vi "MonitoreoSerialDeFlujo.vi"() -> ()   [LabVIEW 2015]
doc: "This VI will continuously monitor the serial port and extract the temperature reading from the received string. This is stored in an array and displayed on the Graph. Press STOP to close the serial port and end the program.\n\nThis program is designed to work with the May 2009 version of the Arduino Temperature program which sends a header, the raw A/D value and the temperature as a float text value.\n\nSelect the appropriate COM port before running this VI. Leave the other serial port settings at their default values (9600, 8, none, 1.0, none)."
uses:
  <vilib>/Instr/_visa.llb/VISA Configure Serial Port (Instr).vi
  <vilib>/MakerHub/LINX/LMH-LINX.lvlib
panel:
  in  "Tiempo de Muestreo":string(combo)
  in  "BaudRate":i32(ring)=10 items=["9600"=9600, "19200"=19200, "38400"=38400, "57600"=57600, "74880"=74880, "115200"=115200]
  in  "Jump Button 4":bool
  in  "Guardar datos a excel":bool
  in  "Rango de grafica":i16(knob) scale=0.0..100.0
  out "FLUJO DE ENTRADA":i32 caption="L/min."
  out "Flujo de entrada y salida":cluster{dbl[], dbl[]}[](graph)
  out "TIEMPO DE MUESTREO":dbl caption="s"
  in  "Jump Button 3":bool
  out "VOLUMEN 1 (L)":i32 caption="L"
  in  "Puerto":refnum<visa-resource-name>="COM3"
  in  "stop":bool
  # "MONITOREO DE SENSORES DE FLUJO YF-S201"
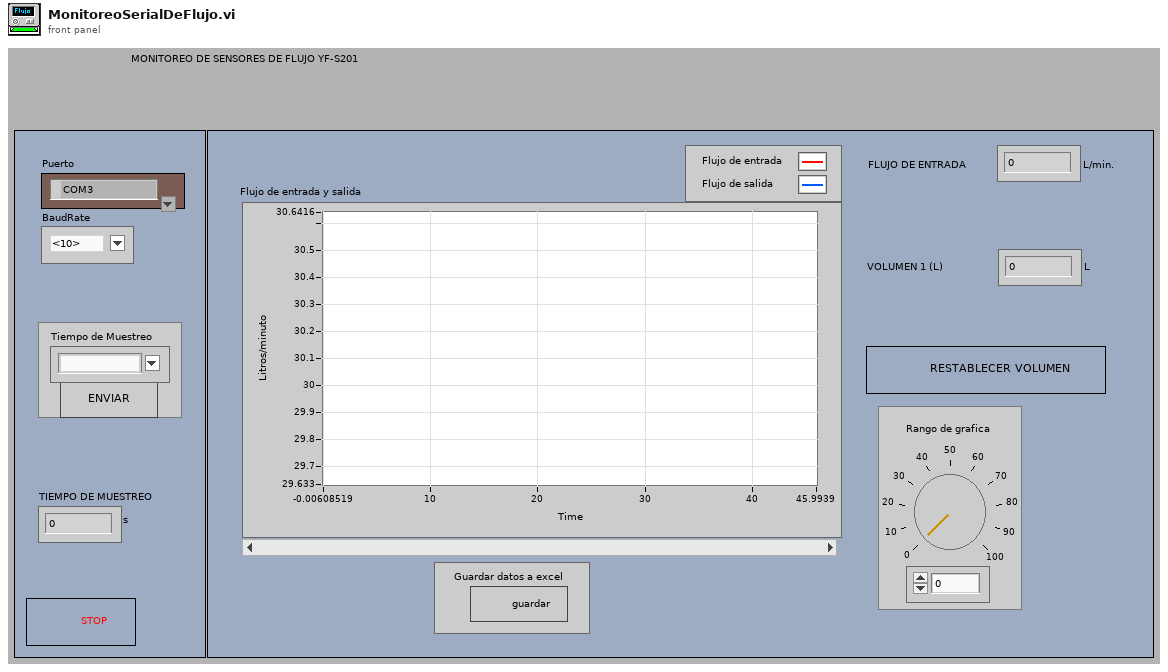
[diagram p1: front panel]
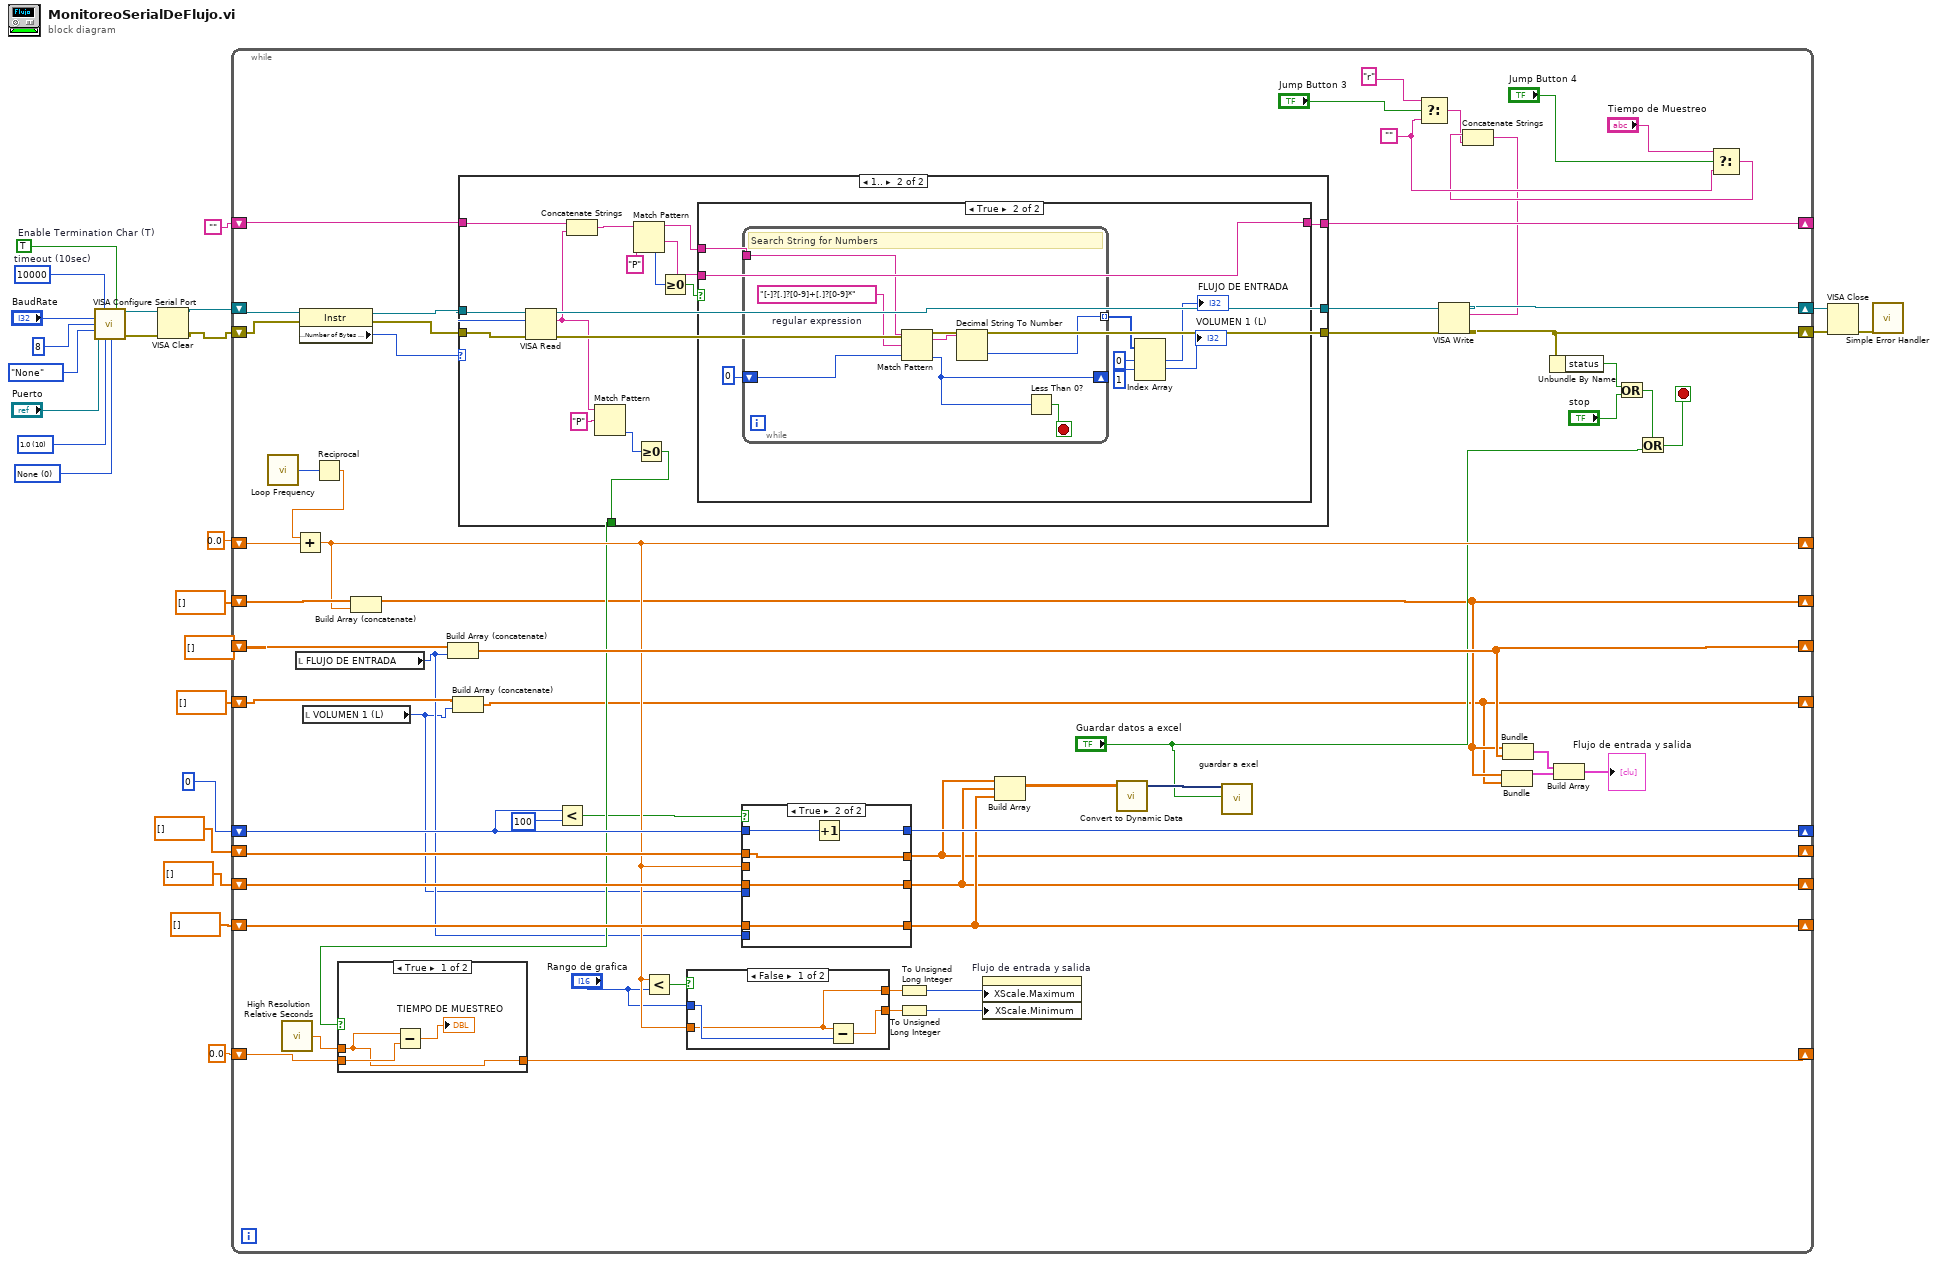
[diagram p0: block diagram]
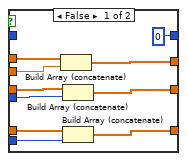
[diagram p2: hidden frame]
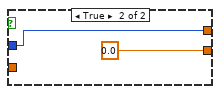
[diagram p3: hidden frame]
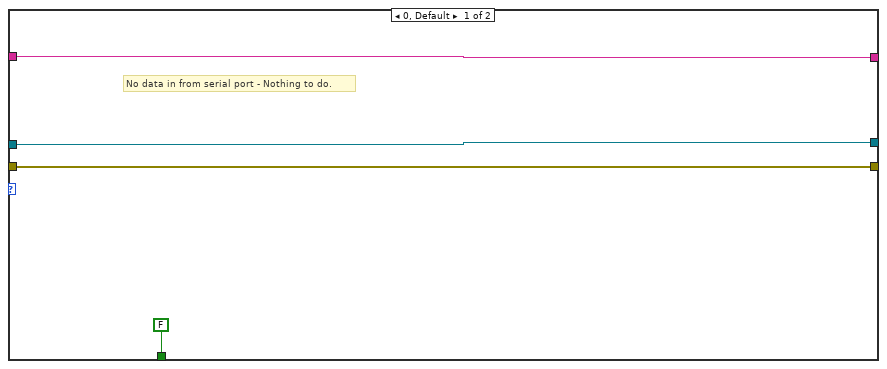
[diagram p5: hidden frame]
diagram:
  w16 = u16 10 items=["1.0"=10, "1.5"=15, "2.0"=20] ("stop bits (10: 1 bit)")
  w17 = u16 0 items=["None", "XON/XOFF", "RTS/CTS", "XON/XOFF & RTS/CTS", "DTR/DSR", "XON/XOFF & DTR/DSR"] ("flow control (0:none)")
  w22 = TRUE  # Enable Termination Char (T)
  w23 = u32 10000  # timeout (10sec)
  n1 = call-poly "VISA Configure Serial Port"("VISA resource name"="Puerto", "timeout (10sec)"=w23, "Enable Termination\nChar (T)"=w22, "baud rate (9600)"="BaudRate", "data bits (8)"=u16 8 ("Data bits (8)"), "parity (0:none)"=enum16{"None", "Odd", "Even", "Mark", "Space"}."None" ("Parity (0:none)"), "stop bits (10: 1 bit)"=w16, "flow control (0:none)"=w17) -> ("VISA resource name out"=w20:refnum<visa-resource-name>, "error out"=w21:errorcluster)  [unwired: 6 in]
  n2 = VISA Clear(VISA resource name=w20, error in (no error)=w21) -> (VISA resource name out=w19:refnum<visa-resource-name>, error out=w3:errorcluster)
  n3 = while {
    shift-right: [w79] -> _
    shift-left: "" -> [w82]
    shift-right: [w27] -> _
    shift-left: dbl[] [] -> [w73]
    shift-right: [w50] -> _
    shift-left: 0.0 -> [w74]
    shift-right: [w61] -> _
    shift-left: dbl[] [] -> [w71]
    shift-right: [w26] -> _
    shift-left: dbl[] [] -> [w72]
    shift-right: [w69] -> _
    shift-left: 0.0 ("relative seconds") -> [w70]
    shift-right: [w56] -> _
    shift-left: 0 -> [w57]
    shift-right: [w51] -> _
    shift-left: dbl[] [] -> [w54]
    shift-right: [w52] -> _
    shift-left: dbl[] [] -> [w53]
    shift-right: [w49] -> _
    shift-left: dbl[] [] -> [w55]
    shift-right: [w76] -> w25
    shift-left: w3 -> [w44]
    shift-right: [w43] -> w2
    shift-left: w19 -> [w84]
    stop <- w60 stop-if-true
    w41 = ""
    n4 = call <vilib>:"Loop Frequency.vi"() -> ("Loop Rate (Hz)"=w64:u32)
    n5 = call <vilib>:"High Resolution Relative Seconds.vi"() -> ("relative seconds"=w65:dbl)
    n6 = local read "FLUJO DE ENTRADA"() -> (w42:i32)
    n7 = property class="Instr"(reference=w84, error in=w44) -> (reference out=w86:refnum<visa-resource-name>, error out=w85:errorcluster, "Serial Settings:Number of Bytes at Serial Port"=w83:u32)
    n8 = local read "VOLUMEN 1 (L)"() -> (w28:i32)
    n9 = Reciprocal(x=w64) -> (1/x=w68:dbl)
    n10 = Add(x=w68, y=w74) -> (x+y=w50:dbl)
    n11 = Build Array (concatenate)(w73, w50) -> (w27:dbl[])
    n12 = Build Array (concatenate)(w71, w42) -> (w61:dbl[])
    n13 = Build Array (concatenate)(w72, w28) -> (w26:dbl[])
    n14 = case shown="1.." w83 {
      selector: w83 -> [_ w126]
      tunnel: [w113 w131] -> w77
      tunnel: [w114 w130] -> w78
      tunnel: w86 -> [w114 w129]
      tunnel: w85 -> [w113 w128]
      tunnel: w82 -> [w112 w127]
      tunnel: [w112 w121] -> w79
      tunnel: [FALSE w115] -> w45
      frame 0, Default {
        # "No data in from serial port - Nothing to do."
      }
      frame 1.. {
        n15 = VISA Read(VISA resource name=w129, byte count=w126, error in (no error)=w128) -> (VISA resource name out=w130:refnum<visa-resource-name>, read buffer=w117:string, error out=w131:errorcluster)  [unwired: 1 out]
        n16 = Concatenate Strings(w127, w117) -> (w120:string)
        n17 = Match Pattern(string=w117, regular expression="P") -> (offset past match=w116:i32)  [unwired: 1 in, 3 out]
        n18 = Match Pattern(string=w120, regular expression="P") -> (before substring=w119:string, after substring=w122:string, offset past match=w124:i32)  [unwired: 1 in, 1 out]
        n19 = Greater Or Equal To 0?(x=w116) -> (x >= 0?=w115:bool)
        n20 = Greater Or Equal To 0?(x=w124) -> (x >= 0?=w123:bool)
        n21 = case shown="True" w123 {
          tunnel: w122 -> [_ w140]
          tunnel: [w132 w140] -> w121
          tunnel: w119 -> [w132 w138]
          frame False {
          }
          frame True {
            n22 = while {
              shift-left: 0 -> [w145]
              shift-right: [w143] -> _
              tunnel: [w147] -> w135 mode=indexing
              tunnel: w138 -> [w141]
              stop <- w146 stop-if-true
              w142 = "[-]?[.]?[0-9]+[.]?[0-9]*"  # regular expression
              # "Search String for Numbers"
              n23 = Match Pattern(string=w141, regular expression=w142, offset (0)=w145) -> (match substring=w144:string, offset past match=w143:i32)  [unwired: 2 out]
              n24 = Decimal String To Number(string=w144) -> (number=w147:i32)  [unwired: 2 in, 1 out]
              n25 = Less Than 0?(x=w143) -> (x < 0?=w146:bool)
            }
            n26 = Index Array(array=w135, index #1=0 ("index"), index #2=1 ("index")) -> (element #1=→"FLUJO DE ENTRADA":i32, element #2=→"VOLUMEN 1 (L)":i32)  [unwired: 1 in, 1 out]
          }
        }
      }
    }
    n27 = case shown="True" w45 {
      tunnel: w70 -> [w109 w110]
      tunnel: w65 -> [w107 _]
      tunnel: [w107 w110] -> w69
      frame True {
        n28 = Subtract(x=w107, y=w109) -> (x-y=→"TIEMPO DE MUESTREO":dbl)
      }
      frame False {
      }
    }
    n29 = Less?(x=w57, y=u32 100) -> (x < y?=w29:bool)
    n30 = Less?(x=w50, y="Rango de grafica") -> (x < y?=w63:bool)
    n31 = case shown="False" w63 {
      tunnel: "Rango de grafica" -> [w103 w105]
      tunnel: [w102 w105] -> w34
      tunnel: [w104 0.0] -> w32
      tunnel: w50 -> [w102 _]
      frame False {
        n32 = Subtract(x=w102, y=w103) -> (x-y=w104:dbl)
      }
      frame True {
      }
    }
    n33 = case shown="True" w29 {
      tunnel: w57 -> [_ w101]
      tunnel: [u32 0 w100] -> w56
      tunnel: w55 -> [w95 w97]
      tunnel: w28 -> [w93 _]
      tunnel: [w96 w99] -> w51
      tunnel: w54 -> [w94 w99]
      tunnel: w42 -> [w91 _]
      tunnel: w53 -> [w92 w98]
      tunnel: [w90 w98] -> w52
      tunnel: [w89 w97] -> w49
      tunnel: w50 -> [w88 _]
      frame False {
        n34 = Build Array (concatenate)(w95, w88) -> (w89:dbl[])
        n35 = Build Array (concatenate)(w94, w93) -> (w96:dbl[])
        n36 = Build Array (concatenate)(w92, w91) -> (w90:dbl[])
      }
      frame True {
        n37 = Increment(x=w101) -> (x+1=w100:u32)
      }
    }
    n38 = To Unsigned Long Integer(number=w34) -> (unsigned 32bit integer=w33:u32)
    n39 = To Unsigned Long Integer(number=w32) -> (unsigned 32bit integer=w31:u32)
    n40 = property on="Flujo de entrada y salida" class="XYGraph (strict)"("XScale.Maximum"=w33, "XScale.Minimum"=w31) -> ()  [unwired: 2 in, 2 out]
    n41 = Build Array(w49, w51, w52) -> (w47:dbl[][])
    n42 = call "Convert to Dynamic Data"("2D Array"=w47) -> ("Dynamic Data Type"=w48:dynamicdata)  [unwired: 3 in]
    n43 = call "guardar a exel"("Signals"=w48, "Enable"="Guardar datos a excel") -> ()  [unwired: 15 in, 3 out]
    n44 = Select(t="r", s="Jump Button 3", f=w41) -> (s? t:f=w38:string)
    n45 = Bundle(w27, w26) -> (w66:cluster{dbl[], dbl[]})  [unwired: 1 in]
    n46 = Bundle(w27, w61) -> (w67:cluster{dbl[], dbl[]})  [unwired: 1 in]
    n47 = Build Array(w67, w66) -> (→"Flujo de entrada y salida":cluster{dbl[], dbl[]}[])
    n48 = Select(t="Tiempo de Muestreo", s="Jump Button 4", f=w41) -> (s? t:f=w39:string)
    n49 = Concatenate Strings(w39, w38) -> (w36:string)
    n50 = VISA Write(VISA resource name=w78, write buffer=w36, error in (no error)=w77) -> (VISA resource name out=w43:refnum<visa-resource-name>, error out=w76:errorcluster)  [unwired: 1 out]
    n51 = Unbundle By Name(w76) -> ("status"=w81:bool)
    n52 = Or(x=w81, y="stop") -> (x .or. y?=w59:bool)
    n53 = Or(x=w59, y="Guardar datos a excel") -> (x .or. y?=w60:bool)
  }
  n54 = VISA Close(VISA resource name=w2, error in (no error)=w25) -> (error out=w24:errorcluster)
  n55 = call <vilib>:"Simple Error Handler.vi"("error in (no error)"=w24) -> ()  [unwired: 4 in, 5 out]
